vi "Prueba.vi"() -> ()   [LabVIEW 2016]
panel:
  in  "D":bool
  in  "C":bool
  in  "B":bool
  in  "A":bool
  out "A0":bool
  out "A1":bool
  out "A2":bool
  out "A3":bool
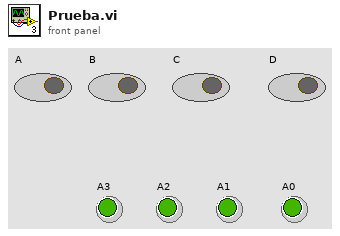
[diagram p1: front panel]
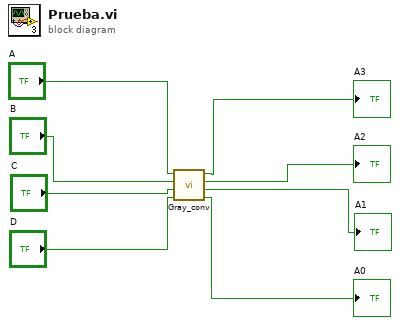
[diagram p0: block diagram]
diagram:
  n1 = call "Gray_conv.vi"("D"="D", "C"="C", "B"="B", "A"="A") -> ("A0"=→"A0":bool, "A1"=→"A1":bool, "A2"=→"A2":bool, "A3"=→"A3":bool)
